vi "VISA.vi"() -> ()   [LabVIEW 2025]
panel:
  out "Instruments":string[](array[string])
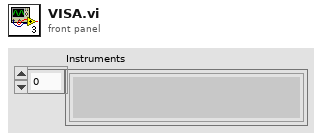
[diagram p1: front panel]
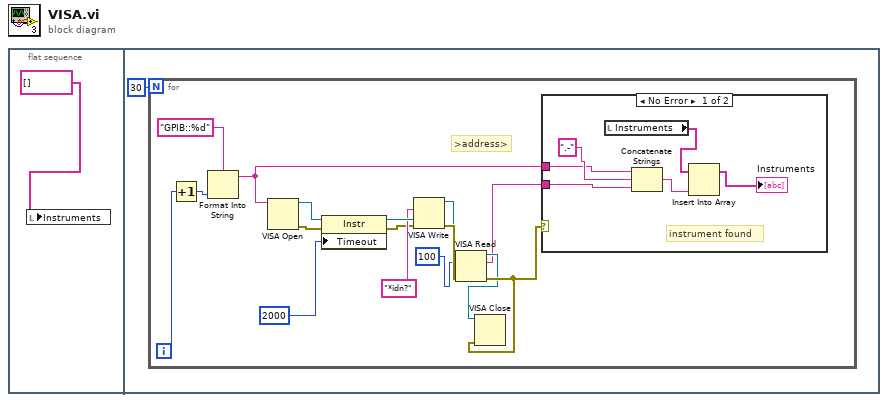
[diagram p0: block diagram]
diagram:
  n1 = flat-sequence {
    frame #0 {
      n2 = local write "Instruments"(string[] []) -> ()
    }
    frame #1 {
      n3 = for {
        N: 30 -> [_]
        i -> [w18]
        # ">address>"
        n4 = Increment(x=w18) -> (x+1=w17:i32)
        n5 = Format Into String(format string="GPIB::%d", w17) -> (resulting string=w15:string)  [unwired: 2 in, 1 out]
        n6 = VISA Open(VISA resource name=w15) -> (VISA resource name=w14:refnum<visa-resource-name>, error out=w13:errorcluster)  [unwired: 4 in]
        n7 = property class="Instr"(reference=w14, error in=w13, "Timeout"=2000) -> (reference out=w12:refnum<visa-resource-name>, error out=w10:errorcluster)
        n8 = VISA Write(VISA resource name=w12, write buffer="*idn?", error in (no error)=w10) -> (VISA resource name out=w7:refnum<visa-resource-name>, error out=w9:errorcluster)  [unwired: 1 out]
        n9 = VISA Read(VISA resource name=w7, byte count=100, error in (no error)=w9) -> (VISA resource name out=w6:refnum<visa-resource-name>, read buffer=w5:string, error out=w8:errorcluster)  [unwired: 1 out]
        n10 = VISA Close(VISA resource name=w6, error in (no error)=w8) -> ()  [unwired: 1 out]
        n11 = case shown="No Error" w8 {
          tunnel: w15 -> [w21 _]
          tunnel: w5 -> [w20 _]
          frame No Error {
            # "instrument found"
            n12 = local read "Instruments"() -> (w19:string[])
            n13 = Concatenate Strings(w21, ".-", w20) -> (w23:string)
            n14 = Insert Into Array(array=w19, new element=w23) -> (→"Instruments":string[])  [unwired: 1 in]
          }
          frame Error {
          }
        }
      }
    }
  }
